vi "Receive Status String.vi"(8 "error in (no error)":errorcluster, 10 "Status String":string, 11 "Operator UI in":refnum<class "Controller UI.lvclass">) -> (0 "error out":errorcluster, 3 "Operator UI out":refnum<class "Controller UI.lvclass">)   [LabVIEW 2016, in "Controller UI.lvlib" / "Controller UI.lvclass"]
uses:
  <userlib>/Common Components/Controller UI/Controller UI.lvclass
  <userlib>/Common Components/Controller UI/Controller UI.lvclass/Controller UI.ctl
  <userlib>/Common Components/Controller UI/Accessors/Read Status Display.vi
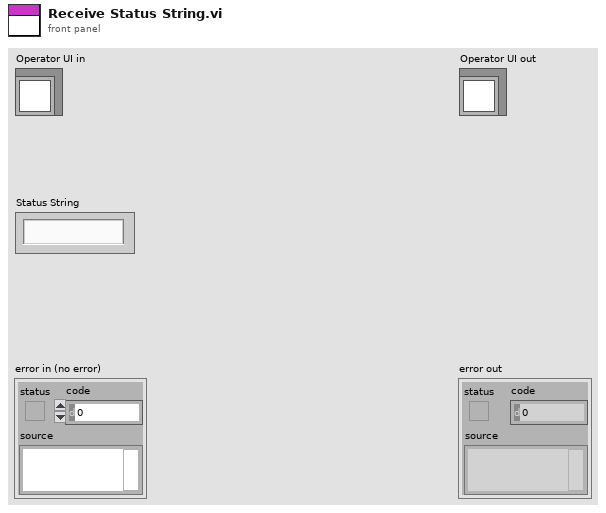
[diagram p1: front panel]
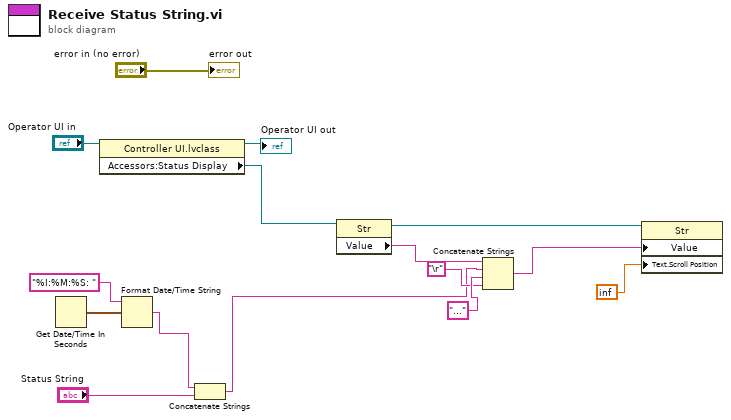
[diagram p0: block diagram]
diagram:
  n1 = Get Date/Time In Seconds() -> (seconds since 1Jan1904=w5:timestamp)
  n2 = property class="Controller UI.lvclass"(reference="Operator UI in") -> (reference out=→"Operator UI out":refnum<class "Controller UI.lvclass">, "Accessors:Status Display"=w1:refnum<vi>)  [unwired: 1 in, 1 out]
  n3 = Format Date/Time String(time format string (%c)="%I:%M:%S: ", seconds (now)=w5) -> (date/time string=w3:string)  [unwired: 1 in]
  n4 = Concatenate Strings(w3, "Status String") -> (w6:string)
  n5 = property class="Str"(reference=w1) -> (reference out=w14:refnum<vi>, "Value"=w13:string)  [unwired: 1 in, 1 out]
  n6 = Concatenate Strings(w13, w6, "..." ("string"), "\r") -> (w12:string)
  n7 = property class="Str"(reference=w14, "Value"=w12, "Text.Scroll Position"=inf) -> ()  [unwired: 1 in, 2 out]
  "error out" <- "error in (no error)"
